vi "FIB spot PXIe-6124.vi"(6 "Z center":dbl=-0.98 min=-1.0 max=1.0, 7 "X center":dbl=-0.98 min=-1.0 max=1.0, 8 "FIB Scan Parameters":T1={"X resolution"=512, "Z resolution"=512, "X center"=0.0, "Z center"=0.0, "X size (V)"=20.0, "Z size (V)"=20.0, "Frame line rampdown ratio"=-0.1, "Scan rate (Hz)"=2000000, "Oversampling"=2} {"Z size (V)" min=0.0 max=20.0; "X size (V)" min=0.0 max=20.0; "Frame line rampdown ratio" min=-1.0 max=1.0 step=0.05 format="%.2g"; "Scan rate (Hz)" max=4000000 format="%#.6p"; "Z resolution" max=2048; "X resolution" max=2048}, 9 "ActiveX Container":refnum<k7>(container), 10 "Options":cluster{"Flip x":bool, "Flip z":bool}={"Flip x"=TRUE, "Flip z"=TRUE}, 11 "HW Config":T2={"FIB X coil"="PXI1Slot7/ao0", "FIB Y coil"="PXI1Slot7/ao1", "Beam blank"="PXI1Slot7/port0/line0", "Ext scan"="PXI1Slot7/port0/line0", "Detector"="PXI1Slot7/ai0", "Shutter Drive"="PXI1Slot2/ao0"}) -> (0 "error out":errorcluster)   [LabVIEW 2018]
uses:
  <vilib>/DAQmx/write.llb/DAQmx Write (Analog 2D DBL NChan NSamp).vi
  <vilib>/DAQmx/create/channels.llb/DAQmx Create Channel (AO-Voltage-Basic).vi
  <vilib>/DAQmx/configure/timing.llb/DAQmx Timing (Sample Clock).vi
  <vilib>/DAQmx/miscellaneous.llb/DAQmx Fill In Error Info.vi
  <resource>/objmgr/daqmx.rc
panel:
  out "Low blanked":bool
  in  "Machine Type":u8(ring) items=["Feiss", "NVision", "Jeiss"]
  out "Ext scan":tag
  out "FIB Y coil":tag
  out "FIB X coil":tag
  out "Beam blank":tag
  in  "spot":bool
  # "Scan coils"
  # "Flip"
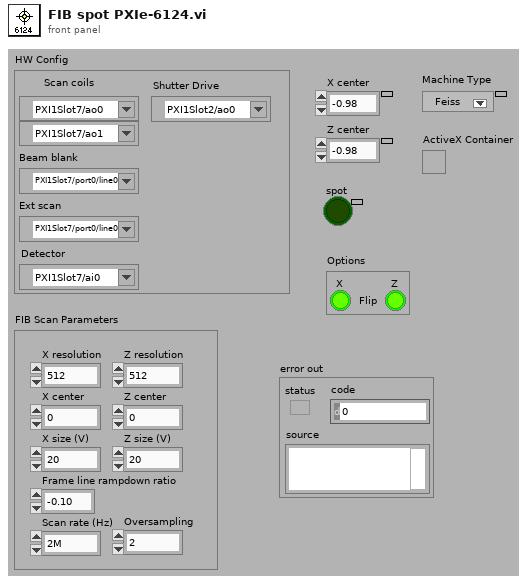
[diagram p1: front panel]
types:
  T1 = cluster{"X resolution":u32, "Z resolution":u32, "X center":dbl, "Z center":dbl, "X size (V)":dbl, "Z size (V)":dbl, "Frame line rampdown ratio":dbl, "Scan rate (Hz)":u32, "Oversampling":u16}
  T2 = cluster{"FIB X coil":tag, "FIB Y coil":tag, "Beam blank":tag, "Ext scan":tag, "Detector":tag, "Shutter Drive":tag}
  T3 = enum16{"SEM", "FIB", "Mill", "SEM + FIB", "Mill + SEM", "Drift SEM", "Drift FIB", "None", "Ext", "Ext + SEM"}
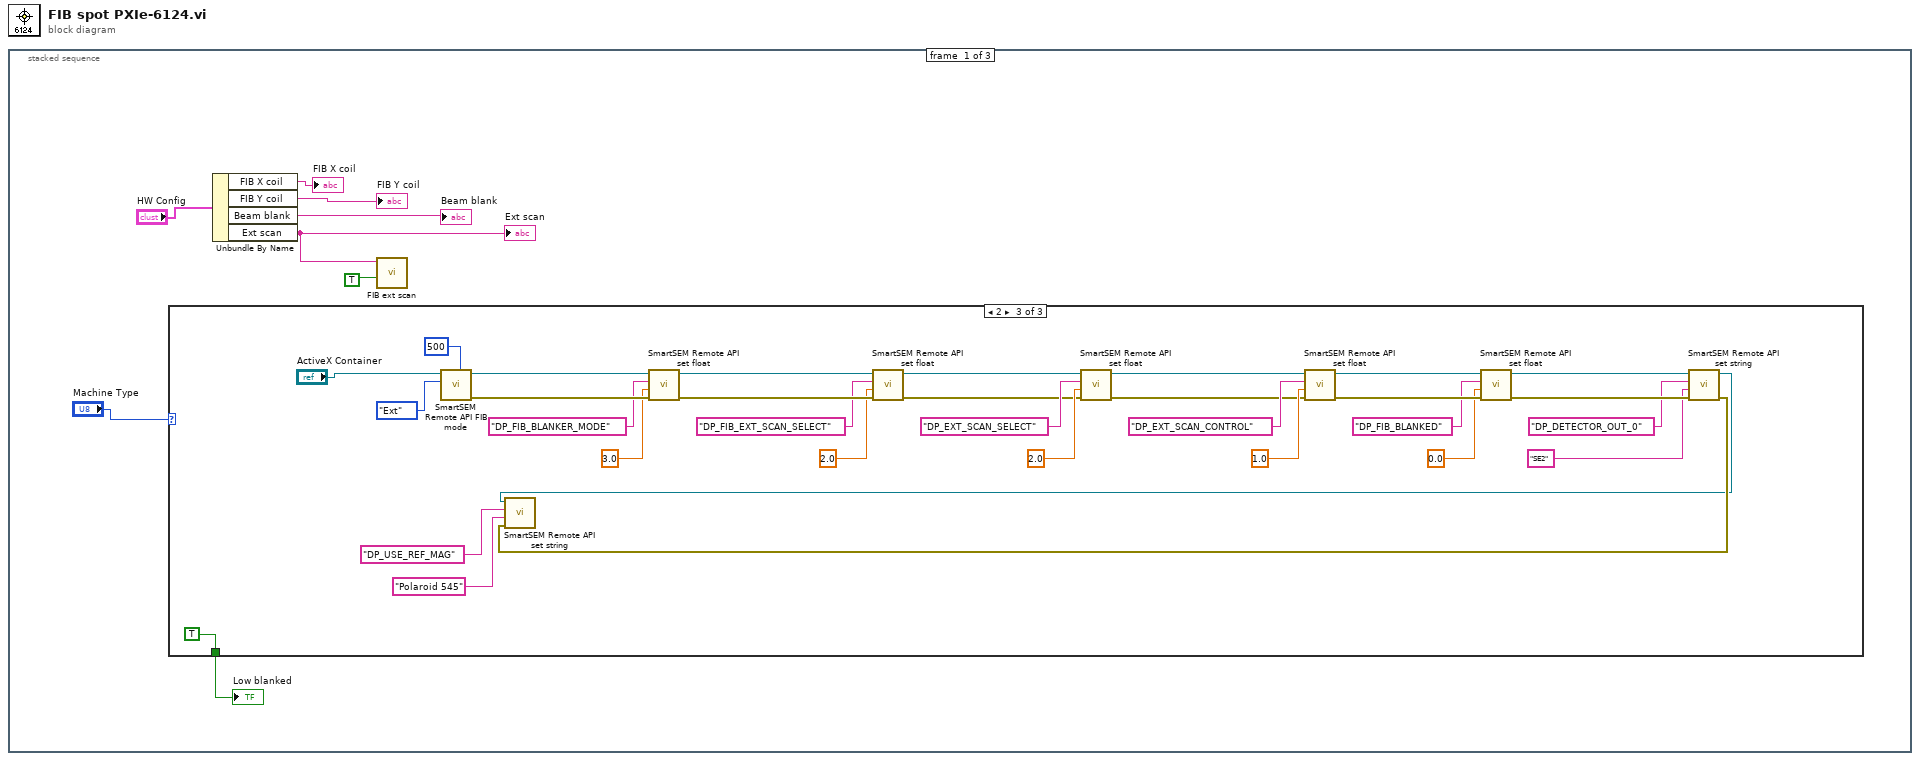
[diagram p0: block diagram]
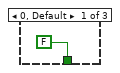
[diagram p2: hidden frame]
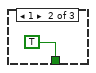
[diagram p3: hidden frame]
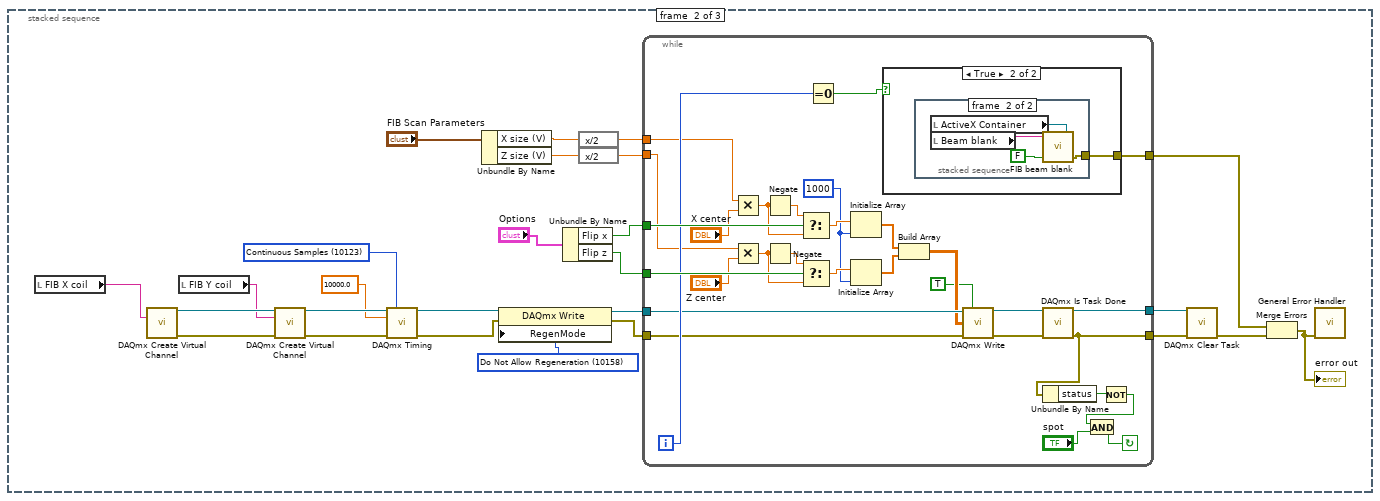
[diagram p4: hidden frame]
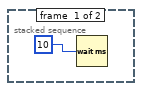
[diagram p6: hidden frame]
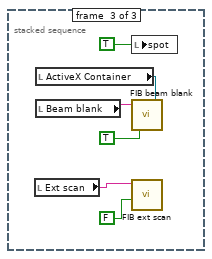
[diagram p7: hidden frame]
diagram:
  n1 = stacked-sequence {
    frame #0 {
      n2 = case shown="2" "Machine Type" {
        tunnel: [FALSE ("Beam blanked") TRUE ("Beam blanked") TRUE ("Beam blanked")] -> w1
        frame 0, Default {
        }
        frame 1 {
        }
        frame 2 {
          n3 = call "SmartSEM Remote API FIB mode.vi"("Wait (ms)"=u32 500, "FIB mode"=T3."Ext", "ActiveX Container"="ActiveX Container") -> ("error out"=w39:errorcluster, "reference out"=w40:refnum<k7>)  [unwired: 7 in]
          n4 = call "SmartSEM Remote API set float.vi"("error in"=w39, "vValue"=sgl 3.0, "lpszParam"="DP_FIB_BLANKER_MODE", "ActiveX Container"=w40) -> ("error out"=w35:errorcluster, "reference out"=w36:refnum<k7>)  [unwired: 6 in]
          n5 = call "SmartSEM Remote API set float.vi"("error in"=w35, "vValue"=sgl 2.0, "lpszParam"="DP_FIB_EXT_SCAN_SELECT" ("lpszCommand"), "ActiveX Container"=w36) -> ("error out"=w13:errorcluster, "reference out"=w14:refnum<k7>)  [unwired: 6 in]
          n6 = call "SmartSEM Remote API set float.vi"("error in"=w13, "vValue"=sgl 2.0, "lpszParam"="DP_EXT_SCAN_SELECT" ("lpszCommand"), "ActiveX Container"=w14) -> ("error out"=w11:errorcluster, "reference out"=w12:refnum<k7>)  [unwired: 6 in]
          n7 = call "SmartSEM Remote API set float.vi"("error in"=w11, "vValue"=sgl 1.0, "lpszParam"="DP_EXT_SCAN_CONTROL" ("lpszCommand"), "ActiveX Container"=w12) -> ("error out"=w29:errorcluster, "reference out"=w30:refnum<k7>)  [unwired: 6 in]
          n8 = call "SmartSEM Remote API set float.vi"("error in"=w29, "vValue"=sgl 0.0, "lpszParam"="DP_FIB_BLANKED", "ActiveX Container"=w30) -> ("error out"=w25:errorcluster, "reference out"=w26:refnum<k7>)  [unwired: 6 in]
          n9 = call "SmartSEM Remote API set string.vi"("error in"=w25, "vValue"="SE2" ("Det A Type"), "lpszParam"="DP_DETECTOR_OUT_0", "ActiveX Container"=w26) -> ("error out"=w17:errorcluster, "reference out"=w16:refnum<k7>)  [unwired: 6 in]
          n10 = call "SmartSEM Remote API set string.vi"("error in"=w17, "vValue"="Polaroid 545" ("lpszParam"), "lpszParam"="DP_USE_REF_MAG", "ActiveX Container"=w16) -> ()  [unwired: 6 in, 2 out]
        }
      }
      "Low blanked" <- w1
      n11 = Unbundle By Name("HW Config") -> ("FIB X coil"=→"FIB X coil":tag, "FIB Y coil"=→"FIB Y coil":tag, "Beam blank"=→"Beam blank":tag, "Ext scan"=w3:tag)
      "Ext scan" <- w3
      n12 = call "FIB ext scan.vi"("Ext on"=TRUE ("data"), "FIB Ext Scan"=w3) -> ()  [unwired: 9 in, 1 out]
    }
    frame #1 {
      w55 = 10123 items=["Finite Samples"=10178, "Continuous Samples"=10123, "Hardware Timed Single Point"=12522] ("sample mode")
      w62 = 10158 items=["Allow Regeneration"=10097, "Do Not Allow Regeneration"=10158] ("RegenMode")
      n13 = local read "FIB X coil"() -> (w57:tag)
      n14 = call-poly <vilib>:"DAQmx Create Virtual Channel.vi"("physical channels"=w57) -> ("task out"=w60:refnum<k21>, "error out"=w61:errorcluster)  [unwired: 8 in, 5 out]
      n15 = local read "FIB Y coil"() -> (w56:tag)
      n16 = call-poly <vilib>:"DAQmx Create Virtual Channel.vi"("task in"=w60, "physical channels"=w56, "error in"=w61) -> ("task out"=w58:refnum<k21>, "error out"=w59:errorcluster)  [unwired: 6 in, 5 out]
      n17 = call-poly <vilib>:"DAQmx Timing.vi"("task/channels in"=w58, "sample mode"=w55, "rate"=10000.0, "error in"=w59) -> ("task out"=w63:refnum<k21>, "error out"=w64:errorcluster)  [unwired: 3 in, 7 out]
      n18 = Unbundle By Name("FIB Scan Parameters") -> ("X size (V)"=w46:dbl, "Z size (V)"=w45:dbl)
      n19 = property class="DAQmx Write"(reference=w63, error in=w64, "RegenMode"=w62) -> (reference out=w52:refnum<k21>, error out=w51:errorcluster)
      n20 = Unbundle By Name("Options") -> ("Flip x"=w65:bool, "Flip z"=w66:bool)
      n21 = expression code="x/2"(w46) -> (w44:dbl)
      n22 = expression code="x/2"(w45) -> (w43:dbl)
      n23 = while {
        tunnel: [w94] -> w67
        tunnel: w66 -> [w91]
        tunnel: w65 -> [w90]
        tunnel: w52 -> [w85]
        tunnel: w51 -> [w84]
        tunnel: [w83] -> w50
        tunnel: [w82] -> w49
        tunnel: w44 -> [w72]
        tunnel: w43 -> [w70]
        i -> [w89]
        stop <- w97 continue-if-true
        w79 = 1000 ("dimension size")
        n24 = Multiply(x=w72, y="X center") -> (x*y=w73:dbl)
        n25 = Multiply(x=w70, y="Z center") -> (x*y=w69:dbl)
        n26 = Negate(x=w73) -> (-x=w93:dbl)
        n27 = Negate(x=w69) -> (-x=w92:dbl)
        n28 = Select(t=w93, s=w90, f=w73) -> (s? t:f=w81:dbl)
        n29 = Select(t=w92, s=w91, f=w69) -> (s? t:f=w80:dbl)
        n30 = Equal To 0?(x=w89) -> (x = 0?=w88:bool)
        n31 = Initialize Array(w81, w79) -> (w78:dbl[])
        n32 = Initialize Array(w80, w79) -> (w77:dbl[])
        n33 = case shown="True" w88 {
          tunnel: [_ w99] -> w94
          frame False {
          }
          frame True {
            n34 = stacked-sequence {
              tunnel: [_ w102] -> w99
              frame #0 {
                n35 = Wait (ms)(milliseconds to wait=u32 10) -> ()  [unwired: 1 out]
              }
              frame #1 {
                n36 = local read "ActiveX Container"() -> (w101:refnum<k7>)
                n37 = local read "Beam blank"() -> (w104:tag)
                n38 = call "FIB beam blank.vi"("ActiveX Container"=w101, "Beam blanked"=FALSE, "lines"=w104) -> ("error out"=w102:errorcluster)  [unwired: 2 in]
              }
            }
          }
        }
        n39 = Build Array(w78, w77) -> (w76:dbl[][])
        n40 = call-poly <vilib>:"DAQmx Write.vi"("task/channels in"=w85, "auto start"=TRUE, "data"=w76, "error in"=w84) -> ("task out"=w86:refnum<k21>, "error out"=w87:errorcluster)  [unwired: 10 out]
        n41 = call <vilib>:"DAQmx Is Task Done.vi"("task/channels in"=w86, "error in"=w87) -> ("task out"=w83:refnum<k21>, "error out"=w82:errorcluster)  [unwired: 2 in, 10 out]
        n42 = Unbundle By Name(w82) -> ("status"=w96:bool)
        n43 = Not(x=w96) -> (.not. x?=w95:bool)
        n44 = And(x=w95, y="spot") -> (x .and. y?=w97:bool)
      }
      n45 = call <vilib>:"DAQmx Clear Task.vi"("task in"=w50, "error in"=w49) -> ("error out"=w48:errorcluster)  [unwired: 13 out]
      n46 = Merge Errors(w67, w48) -> (w68:errorcluster)
      "error out" <- w68
      n47 = call <vilib>:"General Error Handler.vi"("error in (no error)"=w68) -> ()  [unwired: 10 in, 5 out]
    }
    frame #2 {
      n48 = local read "Ext scan"() -> (w107:tag)
      n49 = local read "ActiveX Container"() -> (w105:refnum<k7>)
      n50 = local read "Beam blank"() -> (w109:tag)
      n51 = local write "spot"(TRUE ("stop")) -> ()
      n52 = call "FIB beam blank.vi"("ActiveX Container"=w105, "Beam blanked"=TRUE, "lines"=w109) -> ()  [unwired: 2 in, 1 out]
      n53 = call "FIB ext scan.vi"("Ext on"=FALSE ("data"), "FIB Ext Scan"=w107) -> ()  [unwired: 9 in, 1 out]
    }
  }
